vi "Generate Trace for Skipped Time-Delayed Message.vi"(10 "Delivery Notifier":refnum<notifier>) -> ()   [LabVIEW 2020, in "Actor Framework.lvlib"]
doc: "Generates a DETT User Generated Trace for a repeated time-delayed message deliberately skipping one of its instances."
uses:
  ActorFramework/Time-Delayed Send Message/Time-Delay Override Options.ctl
  Localized Strings.vi
  ActorFramework/Actor Framework.lvlib
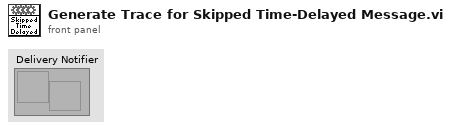
[diagram p1: front panel]
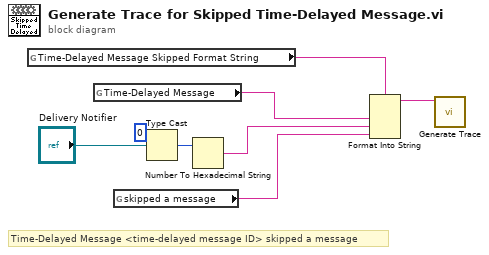
[diagram p0: block diagram]
diagram:
  # "Time-Delayed Message <time-delayed message ID> skipped a message"
  n1 = global read "Localized Strings.vi" "Time-Delayed Message Skipped Format String"() -> (w6:string)
  n2 = global read "Localized Strings.vi" "Time-Delayed Message"() -> (w8:string)
  n3 = global read "Localized Strings.vi" "skipped a message"() -> (w7:string)
  n4 = Type Cast(type=u32 0, x="Delivery Notifier") -> (*(type *) &x=w3:u32)
  n5 = Number To Hexadecimal String(2:w3) -> (0:w2:string)  [unwired: 1 in]
  n6 = Format Into String(format string=w6, w8, w2, w7) -> (resulting string=w1:string)  [unwired: 2 in, 1 out]
  n7 = call "Generate Trace.vi"("String"=w1) -> ()  [unwired: 11 in]
